vi "Build Text Label.vi"(8 "x+y":dbl, 9 "y":dbl, 10 "x":dbl, 11 "Operator":string) -> (3 "Text Label":string)   [LabVIEW 2021]
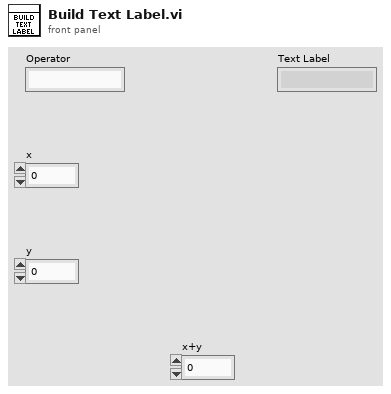
[diagram p1: front panel]
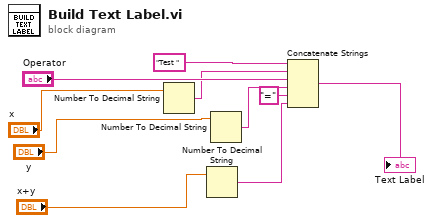
[diagram p0: block diagram]
diagram:
  n1 = Number To Decimal String(number="x") -> (decimal integer string=w4:string)  [unwired: 1 in]
  n2 = Number To Decimal String(number="x+y") -> (decimal integer string=w10:string)  [unwired: 1 in]
  n3 = Number To Decimal String(number="y") -> (decimal integer string=w6:string)  [unwired: 1 in]
  n4 = Concatenate Strings("Test " ("Label"), w4, "Operator", w6, "=" ("chaîne"), w10) -> (→"Text Label":string)
